vi "断电保存全局.vi"() -> ()   [LabVIEW 2016, in "数据传输系统.lvlib"]
panel:
  in  "每日自动重发":bool
  out "参数数值引用":refnum<vi>
  in  "串口透传":bool
  in  "updateconfiguration":T1={"主机"="121.36.219.111", "用户"="std", "密码"="std23506", "远程路径"="UP\\datatransfor\\平台数据传输系统.zip", "下载文件名"="平台数据传输系统.zip", "软件版本"=""}
  in  "STDIP":string[](array[string])=["47.98.43.76", "watersystem", "218.22.44.10", "10.34.1.65", "10.13.3.24"]
  in  "加密传输":bool
  out "剖面数据重发":bool
  out "日志信息重发":bool
  in  "数据重发结束时间":timestamp
  in  "数据重发时间戳":string="1994/10/09 09:20:28"
  out "数据重发":bool
  in  "自动更新":bool=TRUE
  in  "数据库类型":enum16{"Access", "SQLite"}(ring)
  out "data名称":string
  in  "应用环境":T2
  in  "屏蔽维护数据":bool
  in  "数据发送延时时间/s":i32
  in  "判断数据反馈":enum16{"非严格判断", "严格判断", "不判断"}(ring)=enum."严格判断"
  in  "仪器参数发送":bool=TRUE
  in  "地表水/污染源":bool
  in  "暂停上传":bool
  out "等时间间隔分钟":i32
  out "参数系数簇":T3
  out "参数启用数组":bool[](array[boolean])
  out "因子编码簇":T4
  in  "数据触发上传方式":enum16{"出数即刻发送", "间隔时间发送", "整点发送"}(ring)
  in  "系统编码ST":string="21"
  out "配置表格":string[][](table)
  in  "重发时间":T5(ring)
  in  "重发日期":T6(ring)
  in  "每周自动重发":bool=TRUE
  in  "系统编码选择框":string(combo)="地表水质量监测"
  in  "PW":string
  in  "MN":string
  in  "PORT":string
  in  "IP":string
  in  "站点设备":string
  in  "站点名称":string
  in  "baud rate":u32=9600 caption="波特率"
  in  "VISA resource name":refnum<visa-resource-name> caption="VISA资源名称"
  in  "数据发送协议":enum16{"2005-212协议", "2017-212协议"}(ring)=enum."2017-212协议"
  in  "数据发送通道":enum16{"TCP", "VISA"}(ring)
  in  "数据组合发送":bool
  in  "日志、参数发送":bool=TRUE
  in  "2011发送":bool=TRUE
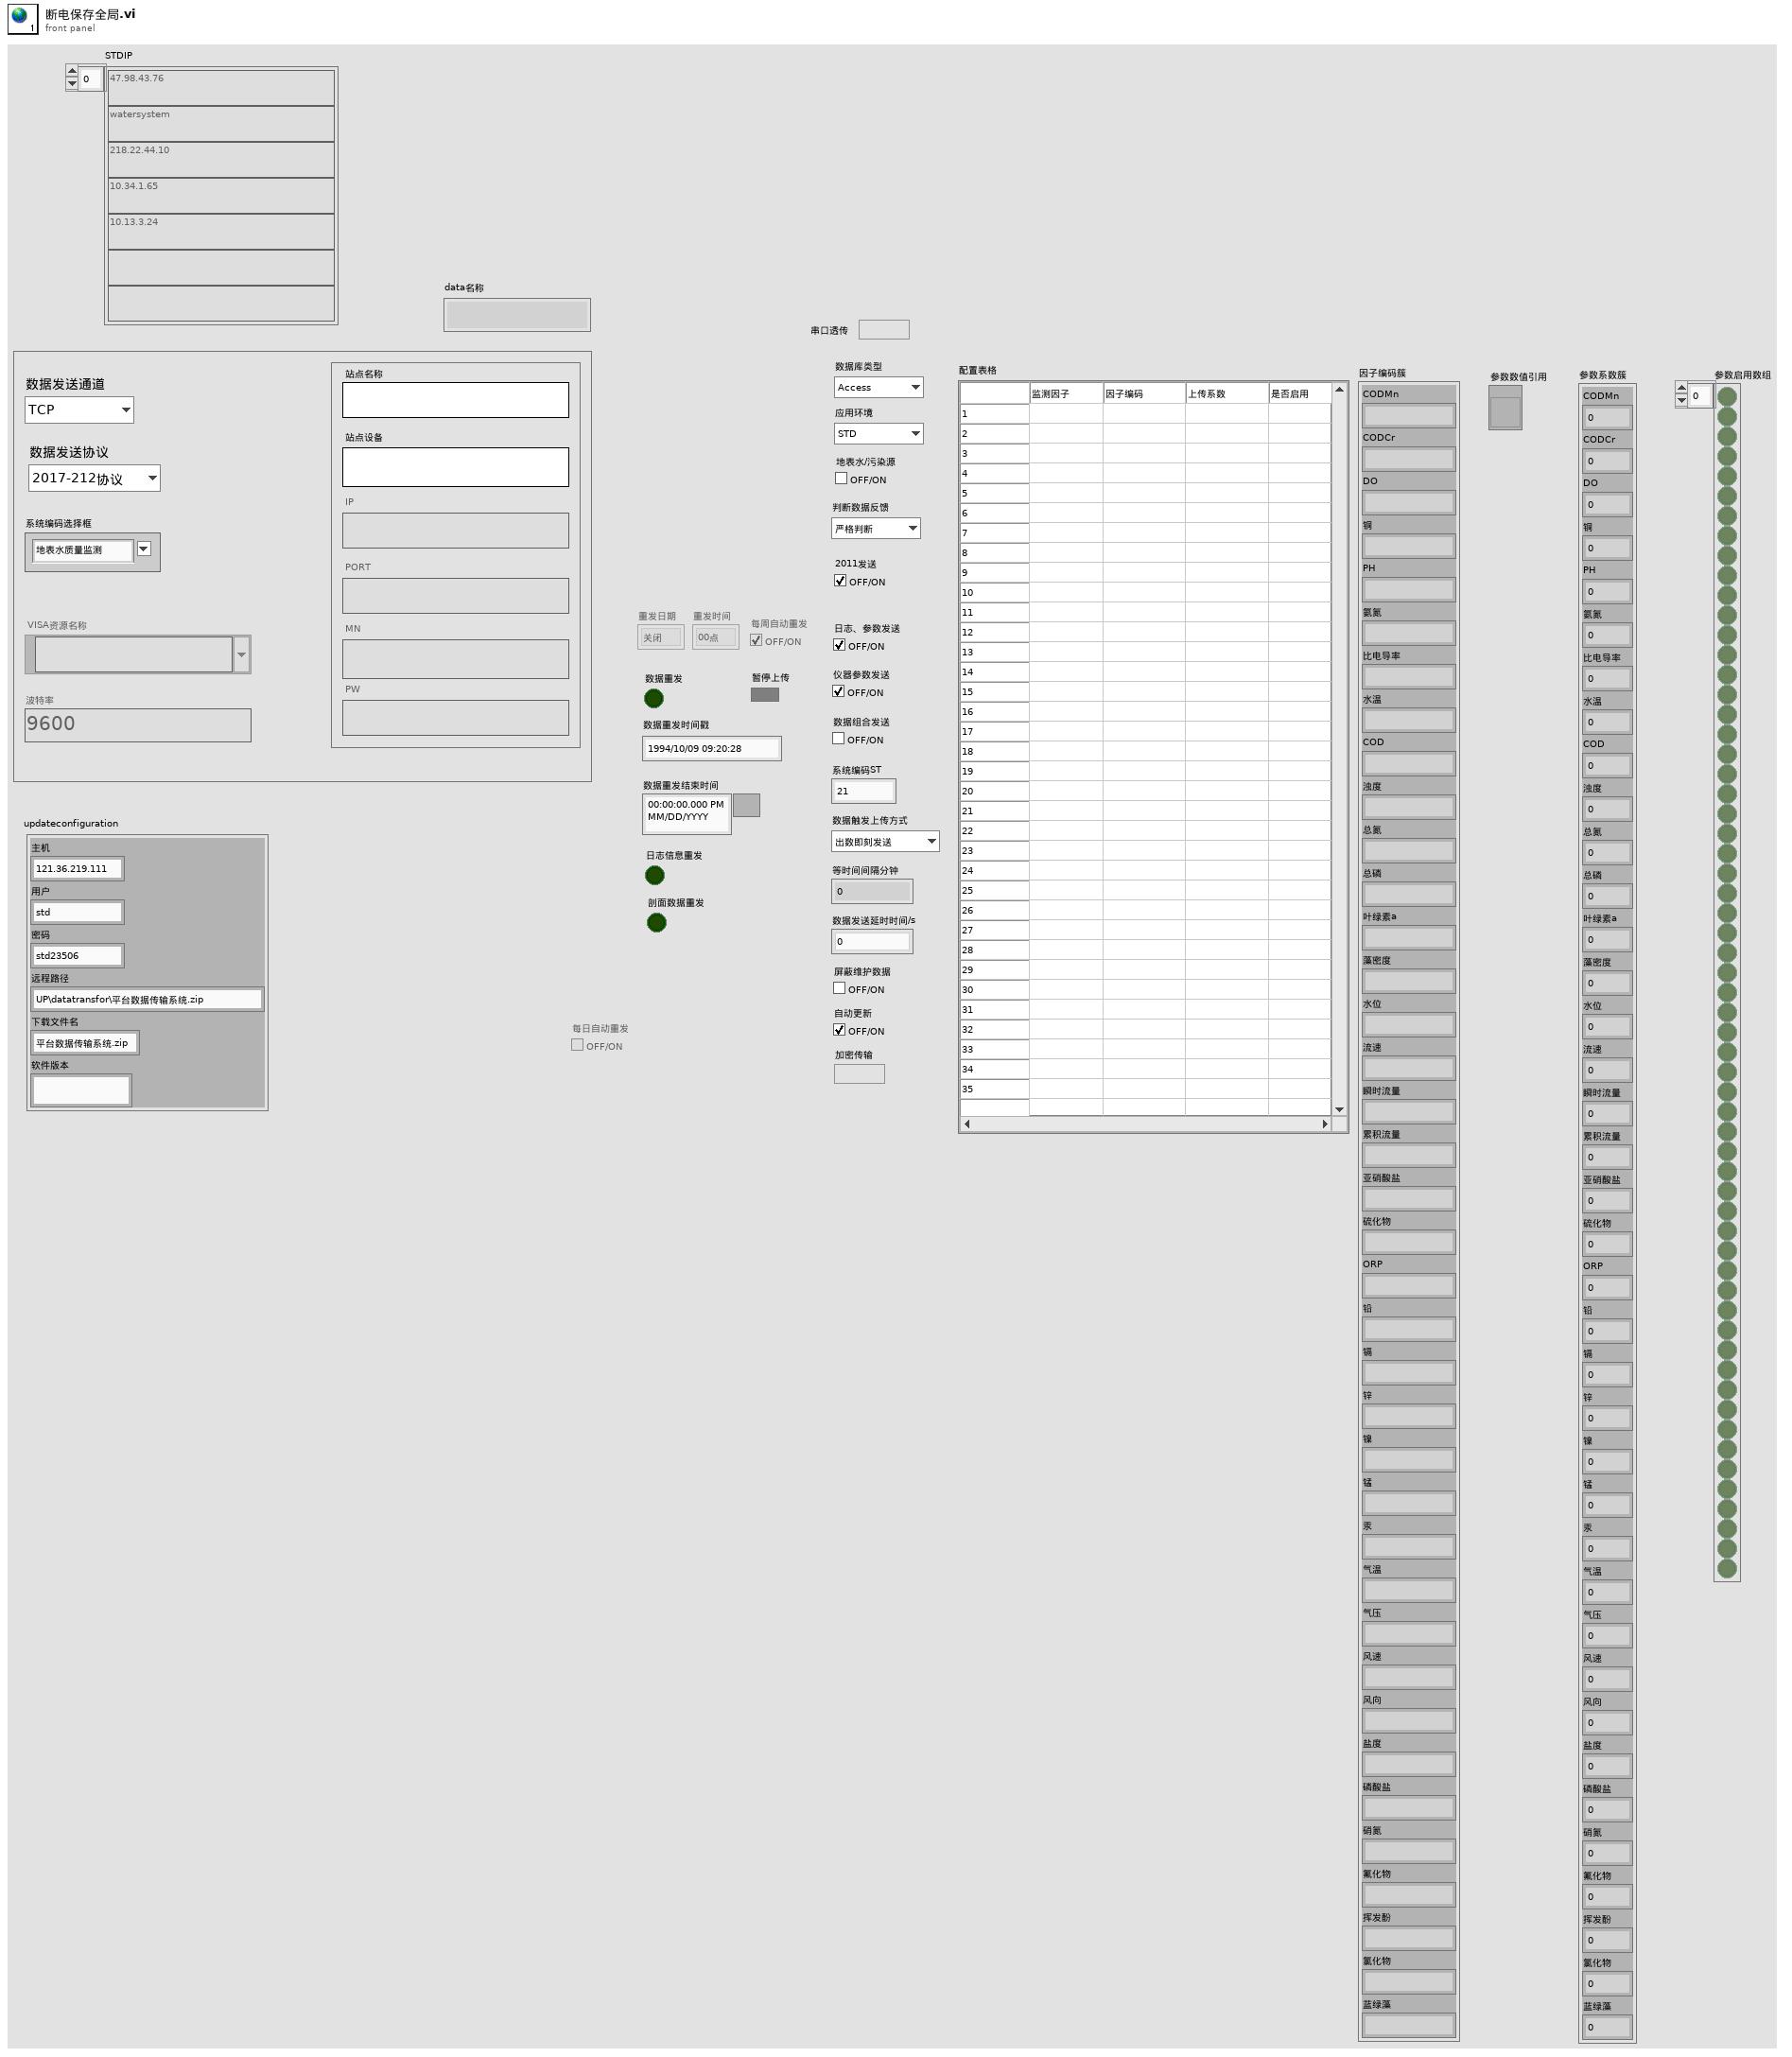
[diagram p1: front panel]
types:
  T1 = cluster{"主机":string, "用户":string, "密码":string, "远程路径":string, "下载文件名":string, "软件版本":string}
  T2 = typedef "数据传输系统.lvlib/应用环境.ctl" = enum16{"STD", "GB212", "婉仪平台"}
  T3 = cluster{"CODMn":dbl, "CODCr":dbl, "DO":dbl, "铜":dbl, "PH":dbl, "氨氮":dbl, "比电导率":dbl, "水温":dbl, "COD":dbl, "浊度":dbl, "总氮":dbl, "总磷":dbl, "叶绿素a":dbl, "藻密度":dbl, "水位":dbl, "流速":dbl, "瞬时流量":dbl, "累积流量":dbl, "亚硝酸盐":dbl, "硫化物":dbl, "ORP":dbl, "铅":dbl, "镉":dbl, "锌":dbl, "镍":dbl, "锰":dbl, "汞":dbl, "气温":dbl, "气压":dbl, "风速":dbl, "风向":dbl, "盐度":dbl, "磷酸盐":dbl, "硝氮":dbl, "氟化物":dbl, "挥发酚":dbl, "氯化物":dbl, "蓝绿藻":dbl}
  T4 = cluster{"CODMn":string, "CODCr":string, "DO":string, "铜":string, "PH":string, "氨氮":string, "比电导率":string, "水温":string, "COD":string, "浊度":string, "总氮":string, "总磷":string, "叶绿素a":string, "藻密度":string, "水位":string, "流速":string, "瞬时流量":string, "累积流量":string, "亚硝酸盐":string, "硫化物":string, "ORP":string, "铅":string, "镉":string, "锌":string, "镍":string, "锰":string, "汞":string, "气温":string, "气压":string, "风速":string, "风向":string, "盐度":string, "磷酸盐":string, "硝氮":string, "氟化物":string, "挥发酚":string, "氯化物":string, "蓝绿藻":string}
  T5 = enum16{"00点", "01点", "02点", "03点", "04点", "05点", "06点", "07点", "08点", "09点", "10点", "11点", "12点", "13点", "14点", "15点", "16点", "17点", "18点", "19点", "20点", "21点", "22点", "23点"}
  T6 = enum16{"关闭", "星期日", "星期一", "星期二", "星期三", "星期四", "星期五", "星期六"}
diagram:
